vi "Set_Rois.vi"(8 "error in":errorcluster, 10 "PicamROI":T1, 11 "camera handle in":u64) -> (0 "error out":errorcluster, 3 "camera handle out":u64)   [LabVIEW 2019, in "PICam.lvlib"]
doc: "Picam_SetParameterRoisValue() configures an Rois parameter to a specified value\nduring camera setup.\n\nIn this VI implementation we only want to specify a single ROI, so the input is a single ROI cluster!"
uses:
  PICam.lvlib
  Ctrls/PicamROI.ctl
  Picam64.dll
panel:
  out "roid":cluster{"roi (U32)":u32, "count (I32)":i32}
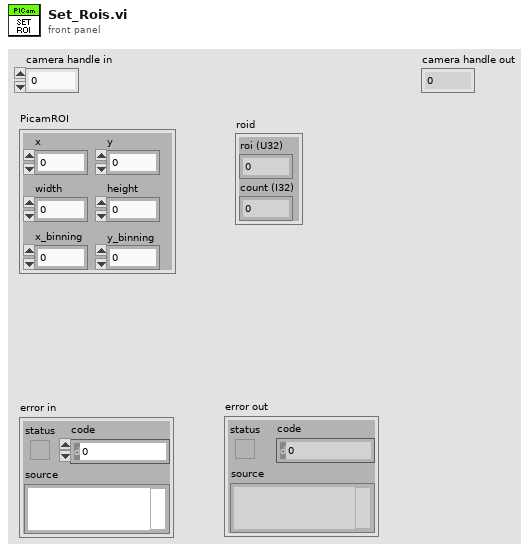
[diagram p1: front panel]
types:
  T1 = typedef "PICam.lvlib/PicamROI.ctl" = cluster{"x":i32, "width":i32, "x_binning":i32, "y":i32, "height":i32, "y_binning":i32}
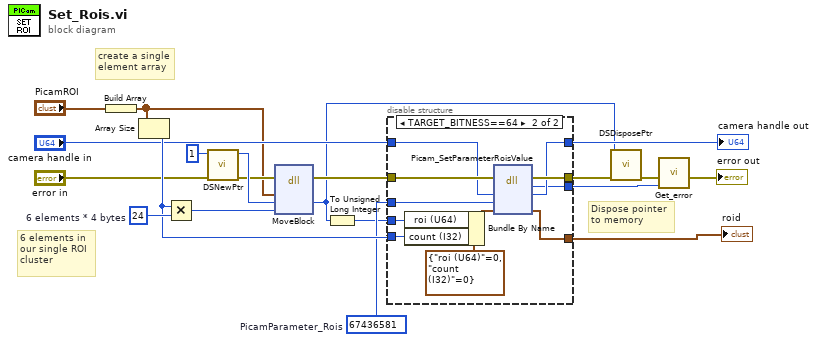
[diagram p0: block diagram]
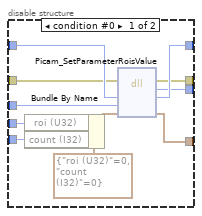
[diagram p2: hidden frame]
diagram:
  w19 = u64 24  # 6 elements * 4 bytes
  w12 = u32 67436581  # PicamParameter_Rois
  # "create a single\nelement array"
  # "6 elements in\nour single ROI\ncluster"
  # "Dispose pointer\nto memory"
  n1 = Build Array("PicamROI") -> (w8:T1[])
  n2 = Array Size(array=w8) -> (size(s)=w15:i32)
  n3 = Multiply(x=w15, y=w19) -> (x*y=w18:u64)
  n4 = call <vilib>:"DSNewPtr.vi"("error in (no error)"="error in", "Size"=u64 1) -> ("error out"=w17:errorcluster, "Pointer"=w20:u64)  [unwired: 8 in]
  n5 = dll-call lib="LabVIEW" fn="MoveBlock"(error in=w17, "src"=w8, "dst"=w20, "size"=w18) -> (error out=w16:errorcluster, "dst"=w7:u64)  [unwired: 5 in, 1 out]
  n6 = To Unsigned Long Integer(number=w7) -> (unsigned 32bit integer=w2:u32)
  n7 = disable-structure shown="TARGET_BITNESS==64" {
    disable-tunnel: "camera handle in" -> [w29 w39]
    disable-tunnel: w2 -> [w25 w37]
    disable-tunnel: w16 -> [w28 w42]
    disable-tunnel: [w27 w38] -> w13
    disable-tunnel: w12 -> [w26 w33]
    disable-tunnel: [w24 w41] -> w14
    disable-tunnel: w15 -> [w23 w36]
    disable-tunnel: [w22 w35] -> w6
    disable-tunnel: [w21 w32] -> w3
    frame condition #0 {
      n8 = Bundle By Name(cluster=cluster{"roi (U32)":u32, "count (I32)":i32} {"roi (U32)"=0, "count (I32)"=0}, "roi (U32)"=w25, "count (I32)"=w23) -> (w30:cluster{"roi (U32)":u32, "count (I32)":i32})
      n9 = dll-call lib="Picam*.*" fn="Picam_SetParameterRoisValue"(error in=w28, "handle"=w29, "param"=w26, "roid"=w30) -> (error out=w24:errorcluster, "return type"=w22:i32, "handle"=w27:u64, "roid"=w21:cluster{"roi (U32)":u32, "count (I32)":i32})  [unwired: 3 in, 1 out]
    }
    frame condition #1 (active) {
      n10 = Bundle By Name(cluster=cluster{"roi (U64)":u64, "count (I32)":u64} {"roi (U64)"=0, "count (I32)"=0}, "roi (U64)"=w37, "count (I32)"=w36) -> (w40:cluster{"roi (U64)":u64, "count (I32)":u64})
      n11 = dll-call lib="Picam*.*" fn="Picam_SetParameterRoisValue"(error in=w42, "handle"=w39, "param"=w33, "roid"=w40) -> (error out=w41:errorcluster, "return type"=w35:i32, "handle"=w38:u64, "roid"=w32:cluster{"roi (U64)":u64, "count (I32)":u64})  [unwired: 3 in, 1 out]
    }
  }
  "camera handle out" <- w13
  "roid" <- w3
  n12 = call <vilib>:"DSDisposePtr.vi"("error in (no error)"=w14, "Pointer"=w7) -> ("error out"=w5:errorcluster)  [unwired: 9 in]
  n13 = call "Get_error.vi"("PICam_Error"=w6, "error in (no error)"=w5) -> ("error out"=→"error out":errorcluster)  [unwired: 9 in]
